vi "RTTrapTest-19-08-2016.vi"() -> ()   [LabVIEW 2010]
uses:
  <vilib>/userDefined/High Color/nirio_resource_hc.ctl
  <vilib>/rvi/interface/nirviOpenFPGA/nirviOpenFPGA.xnode
  C:/Users/HAGAR-IV/Desktop/Zeugs/Johnny/pertrasgc fpga/FPGA-TrapTest-19-08-2016.vi
  <vilib>/rvi/ClientSDK/nirviWhatTheDeviceIsDoing.ctl
  <vilib>/rvi/interface/nirviReadWriteControl/nirviReadWriteControl.xnode
  <vilib>/rvi/interface/common/niFpgaNodeNameForErrorReporting.ctl
  <vilib>/rvi/errors/niLvFpgaWhatHappensToTopLevelVI.ctl
  <vilib>/rvi/interface/nirviMethod/nirviMethod.xnode
  <vilib>/rvi/interface/nirviCloseFPGA/nirviCloseFPGA.xnode
  <vilib>/FPGAPlugInAG/cRIO-9114/niLvFpga_Open_cRIO-9114.vi
  <vilib>/rvi/interface/common/dynamic/niFpgaDynamicAddResources.vi
  <vilib>/Utility/error.llb/Error Cluster From Error Code.vi
  <vilib>/rvi/errors/niLvFpgaAdjustHostInterfaceError.vi
  <vilib>/FPGAPlugInAG/Dynamic/niLvFpga_Close_Dynamic.vi
  NiFpgaLv.dll
panel:
  out "ThermoTemp":dbl
  out "PTTempTrap":dbl[](graph)
  in  "ThermoKoeff0":dbl=12.98
  in  "ThermoKoeff2":dbl=-136.78
  in  "ThermoKoeff1":dbl=1284.53
  in  "PTStirlingKoeff0":dbl=-248.216
  in  "PTStirlingKoeff2":dbl=3.13106
  in  "PTStirlingKoeff1":dbl=103.576
  in  "SollwertTemp":dbl=50.0
  in  "R(T)Koeff0":dbl=6.02
  in  "R(T)Koeff2":dbl=-7.1e-06
  in  "R(T)Koeff1":dbl=0.0264
  out "TempTrap":dbl[](graph)
  in  "Löschen":bool
  out "SollwertSchpannung":dbl
  out "SollwertWidrschtond":dbl=8.43
  out "TempTrap":dbl
  in  "T(R)Koeff0":dbl=-209.4
  in  "T(R)Koeff2":dbl=0.46
  in  "T(R)Koeff1":dbl=32.0
  out "WiderstandHeizdraht":dbl
  out "PTStirling":dbl format="%.2f"
  in  "Stirling":bool
  out "Thermo [V]":fxp<+/-,26,5> format="%.23g"
  in  "Messwerte":i32=10
  in  "Heizen":bool
  in  "5Van(us)":u16=5500
  in  "Periode(us)":u32=100000
  out "Messwert":fxp<+/-,27,6> format="%.23g"
  in  "Warten(us)":u16=5000
  in  "zwischenMesswerten(us)":u16=10
  in  "PID gains":T1={"proportional gain (Kc)"=5.0, "integral gain (Kc*Ts/Ti)"=0.0, "derivative gain (Kc*Td/Ts)"=0.0} {"proportional gain (Kc)" format="%.11g"; "integral gain (Kc*Ts/Ti)" format="%.11g"; "derivative gain (Kc*Td/Ts)" format="%.11g"}
  in  "stop":bool
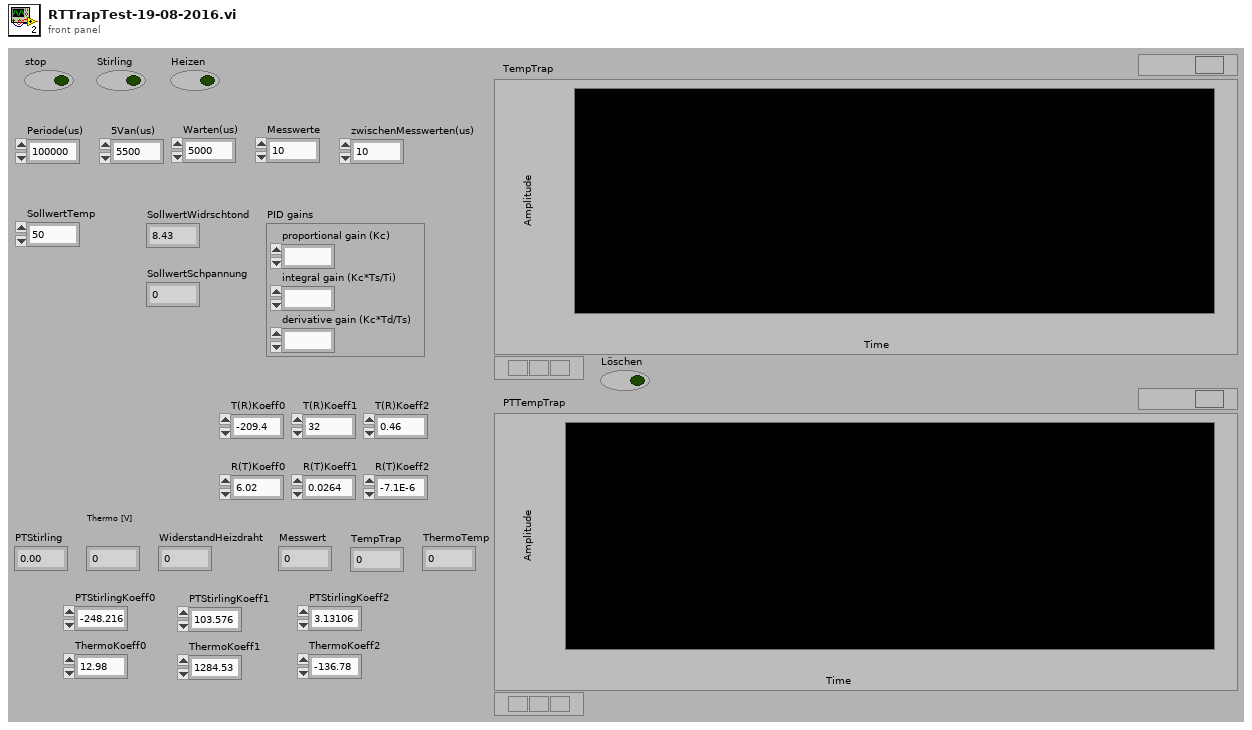
[diagram p1: front panel]
types:
  T1 = cluster{"proportional gain (Kc)":fxp<+/-,16,8>, "integral gain (Kc*Ts/Ti)":fxp<+/-,16,8>, "derivative gain (Kc*Td/Ts)":fxp<+/-,16,8>}
  T2 = typedef "niFpgaNodeNameForErrorReporting.ctl" = enum16{"Open FPGA VI Reference", "Read/Write Control", "Invoke Method: Abort", "Invoke Method: Acknowledge IRQ", "Invoke Method: Download", "Invoke Method: FIFO.Configure", "Invoke Method: FIFO.Read", "Invoke Method: FIFO.Start", "Invoke Method: FIFO.Stop", "Invoke Method: FIFO.Write", "Invoke Method: Reset", "Invoke Method: Run", "Invoke Method: Wait on IRQ", "Close FPGA VI Reference"}
  T3 = typedef "niLvFpgaWhatHappensToTopLevelVI.ctl" = enum16{"top level VI scripted behind XNode", "top level VI inlined behind XNode"}
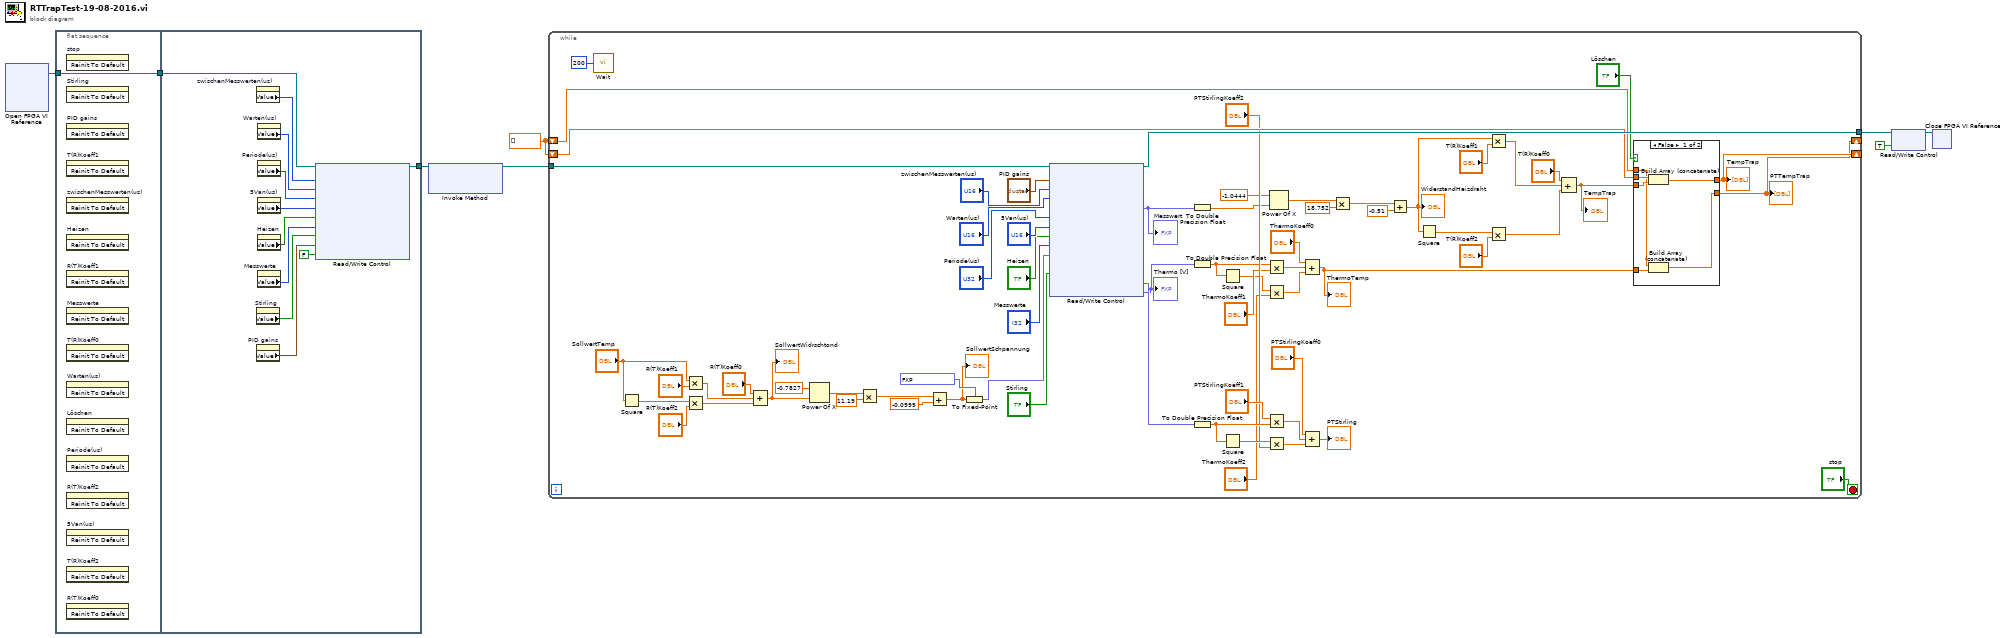
[diagram p0: block diagram]
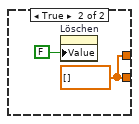
[diagram p2: hidden frame]
diagram:
  w1 = dbl[] []
  n1 = xnode "Open FPGA VI Reference"() -> ("FPGA VI Reference Out"=w8:refnum<k20>)  [unwired: 2 in, 1 out]
  n2 = flat-sequence {
    tunnel: w8 -> [w9]
    tunnel: [w9] -> w2
    tunnel: [w19] -> w7
    tunnel: w2 -> [w20]
    frame #0 {
      n3 = invoke on="stop" class="Bool (strict)" method="Reinit To Default"() -> ()  [unwired: 3 in, 3 out]
      n4 = invoke on="Stirling" class="Bool (strict)" method="Reinit To Default"() -> ()  [unwired: 3 in, 3 out]
      n5 = invoke on="PID gains" class="Clust (strict)" method="Reinit To Default"() -> ()  [unwired: 3 in, 3 out]
      n6 = invoke on="T(R)Koeff1" class="DigNum (strict)" method="Reinit To Default"() -> ()  [unwired: 3 in, 3 out]
      n7 = invoke on="zwischenMesswerten(us)" class="DigNum (strict)" method="Reinit To Default"() -> ()  [unwired: 3 in, 3 out]
      n8 = invoke on="Heizen" class="Bool (strict)" method="Reinit To Default"() -> ()  [unwired: 3 in, 3 out]
      n9 = invoke on="R(T)Koeff1" class="DigNum (strict)" method="Reinit To Default"() -> ()  [unwired: 3 in, 3 out]
      n10 = invoke on="Messwerte" class="DigNum (strict)" method="Reinit To Default"() -> ()  [unwired: 3 in, 3 out]
      n11 = invoke on="T(R)Koeff0" class="DigNum (strict)" method="Reinit To Default"() -> ()  [unwired: 3 in, 3 out]
      n12 = invoke on="Warten(us)" class="DigNum (strict)" method="Reinit To Default"() -> ()  [unwired: 3 in, 3 out]
      n13 = invoke on="Löschen" class="Bool (strict)" method="Reinit To Default"() -> ()  [unwired: 3 in, 3 out]
      n14 = invoke on="Periode(us)" class="DigNum (strict)" method="Reinit To Default"() -> ()  [unwired: 3 in, 3 out]
      n15 = invoke on="R(T)Koeff2" class="DigNum (strict)" method="Reinit To Default"() -> ()  [unwired: 3 in, 3 out]
      n16 = invoke on="5Van(us)" class="DigNum (strict)" method="Reinit To Default"() -> ()  [unwired: 3 in, 3 out]
      n17 = invoke on="T(R)Koeff2" class="DigNum (strict)" method="Reinit To Default"() -> ()  [unwired: 3 in, 3 out]
      n18 = invoke on="R(T)Koeff0" class="DigNum (strict)" method="Reinit To Default"() -> ()  [unwired: 3 in, 3 out]
    }
    frame #1 {
      n19 = property on="zwischenMesswerten(us)" class="DigNum (strict)"() -> ("Value"=w18:u16)  [unwired: 2 in, 2 out]
      n20 = property on="Stirling" class="Bool (strict)"() -> ("Value"=w12:bool)  [unwired: 2 in, 2 out]
      n21 = property on="PID gains" class="Clust (strict)"() -> ("Value"=w11:T1)  [unwired: 2 in, 2 out]
      n22 = property on="Warten(us)" class="DigNum (strict)"() -> ("Value"=w17:u16)  [unwired: 2 in, 2 out]
      n23 = property on="Periode(us)" class="DigNum (strict)"() -> ("Value"=w16:u32)  [unwired: 2 in, 2 out]
      n24 = property on="5Van(us)" class="DigNum (strict)"() -> ("Value"=w15:u16)  [unwired: 2 in, 2 out]
      n25 = property on="Heizen" class="Bool (strict)"() -> ("Value"=w14:bool)  [unwired: 2 in, 2 out]
      n26 = property on="Messwerte" class="DigNum (strict)"() -> ("Value"=w13:i32)  [unwired: 2 in, 2 out]
      n27 = xnode "Read/Write Control"("FPGA VI Reference In"=w20, "zwischenMesswerten(us)"=w18, "Warten(us)"=w17, "Periode(us)"=w16, "5Van(us)"=w15, "Heizen"=w14, "Messwerte"=w13, "Stirling"=w12, "PID gains"=w11, "stop"=FALSE) -> ("FPGA VI Reference Out"=w19:refnum<k20>)  [unwired: 1 in, 1 out]
    }
  }
  n28 = xnode "Invoke Method"("FPGA VI Reference In"=w7) -> ("FPGA VI Reference Out"=w6:refnum<k20>)  [unwired: 2 in, 1 out]
  n29 = while {
    tunnel: w6 -> [w301]
    tunnel: [w299] -> w5
    shift-right: [w277] -> _
    shift-left: w1 -> [w279]
    shift-right: [w251] -> _
    shift-left: w1 -> [w260]
    stop <- "stop" stop-if-true
    n30 = call "Wait"("Count(mSec)"=u32 200) -> ()  [unwired: 1 out]
    n31 = Square(x="SollwertTemp") -> (x^2=w276:dbl)
    n32 = Multiply(x="SollwertTemp", y="R(T)Koeff1") -> (x*y=w271:dbl)
    n33 = Multiply(x=w276, y="R(T)Koeff2") -> (x*y=w270:dbl)
    n34 = Compound Arithmetic op=ADD("R(T)Koeff0", w271, w270) -> (w245:dbl)
    "SollwertWidrschtond" <- w245
    n35 = Power Of X(1:w245, 2:-0.7827 ("y")) -> (0:w241:dbl)
    n36 = Multiply(x=w241, y=11.19) -> (x*y=w239:dbl)
    n37 = Add(x=w239, y=-0.0999) -> (x+y=w237:dbl)
    "SollwertSchpannung" <- w237
    n38 = To Fixed-Point(fixed-point type=fxp<+/-,16,6> 0.0 ("setpoint"), number=w237) -> (fixed-point=w282:fxp<+/-,16,6>)
    n39 = xnode "Read/Write Control"("FPGA VI Reference In"=w301, "PID gains"="PID gains", "zwischenMesswerten(us)"="zwischenMesswerten(us)", "Warten(us)"="Warten(us)", "Periode(us)"="Periode(us)", "5Van(us)"="5Van(us)", "Heizen"="Heizen", "Messwerte"="Messwerte", "setpoint"=w282, "Stirling"="Stirling") -> ("FPGA VI Reference Out"=w299:refnum<k20>, "Messwert"=w284:fxp<+/-,27,6>, "PTStirling"=w262:fxp<+/-,26,5>, "Thermoelement"=w236:fxp<+/-,26,5>)  [unwired: 1 in, 2 out]
    "Messwert" <- w284
    "Thermo [V]" <- w236
    n40 = To Double Precision Float(number=w284) -> (double precision float=w244:dbl)
    n41 = To Double Precision Float(number=w236) -> (double precision float=w256:dbl)
    n42 = To Double Precision Float(number=w262) -> (double precision float=w268:dbl)
    n43 = Square(x=w256) -> (x^2=w255:dbl)
    n44 = Square(x=w268) -> (x^2=w267:dbl)
    n45 = Multiply(x=w256, y="ThermoKoeff1") -> (x*y=w257:dbl)
    n46 = Multiply(x=w255, y="ThermoKoeff2") -> (x*y=w253:dbl)
    n47 = Multiply(x="PTStirlingKoeff1", y=w268) -> (x*y=w264:dbl)
    n48 = Multiply(x=w267, y="PTStirlingKoeff2") -> (x*y=w263:dbl)
    n49 = Power Of X(1:w244, 2:-1.0444 ("x")) -> (0:w250:dbl)
    n50 = Compound Arithmetic op=ADD("ThermoKoeff0", w257, w253) -> (w252:dbl)
    "ThermoTemp" <- w252
    n51 = Compound Arithmetic op=ADD("PTStirlingKoeff0", w264, w263) -> (→"PTStirling":dbl)
    n52 = Multiply(x=w250, y=18.752) -> (x*y=w248:dbl)
    n53 = Add(x=w248, y=-0.51) -> (x+y=w246:dbl)
    "WiderstandHeizdraht" <- w246
    n54 = Square(x=w246) -> (x^2=w289:dbl)
    n55 = Multiply(x=w246, y="T(R)Koeff1") -> (x*y=w286:dbl)
    n56 = Multiply(x=w289, y="T(R)Koeff2") -> (x*y=w287:dbl)
    n57 = Compound Arithmetic op=ADD("T(R)Koeff0", w286, w287) -> (w280:dbl)
    "TempTrap" <- w280
    n58 = case shown="False" "Löschen" {
      tunnel: w280 -> [w307 _]
      tunnel: [w306 w308] -> w277
      tunnel: w279 -> [w305 _]
      tunnel: [w304 w308] -> w251
      tunnel: w260 -> [w303 _]
      tunnel: w252 -> [w302 _]
      frame False {
        n59 = Build Array (concatenate)(w305, w307) -> (w306:dbl[])
        n60 = Build Array (concatenate)(w303, w302) -> (w304:dbl[])
      }
      frame True {
        w308 = dbl[] []
        n61 = property on="Löschen" class="Bool (strict)"("Value"=FALSE ("Löschen")) -> ()  [unwired: 2 in, 2 out]
      }
    }
    "TempTrap" <- w277
    "PTTempTrap" <- w251
  }
  n62 = xnode "Read/Write Control"("FPGA VI Reference In"=w5, "stop"=TRUE) -> ("FPGA VI Reference Out"=w3:refnum<k20>)  [unwired: 1 in, 1 out]
  n63 = xnode "Close FPGA VI Reference"("FPGA VI Reference In"=w3) -> ()  [unwired: 1 in, 1 out]
